vi "Json_Data_Path.vi"(2 "Json File Path":path, 7 "ERD Data Out":cluster{"ERD Number":u16, "Data":string}[](array[cluster]) {"ERD Number" format="%.0x"}, 11 "error in":errorcluster) -> (6 "Array":T1(array[cluster]) {"ERD Number" format="%x"}, 15 "error out":errorcluster)   [LabVIEW 2021]
uses:
  <vilib>/JDP Science/JSONtext/String Subset.vi
  <vilib>/JDP Science/JSONtext/support/Strip Quotes and Unescape.vi
  <vilib>/JDP Science/JSONtext/support/Unescape JSON string.vi
  <vilib>/JDP Science/JSONtext/Parsing/Parse Full Path or Item Name.vi
  <vilib>/JDP Science/JSONtext/Offset/Find Item Locations by Path.vi
  <vilib>/JDP Science/JSONtext/JSONtext.lvlib
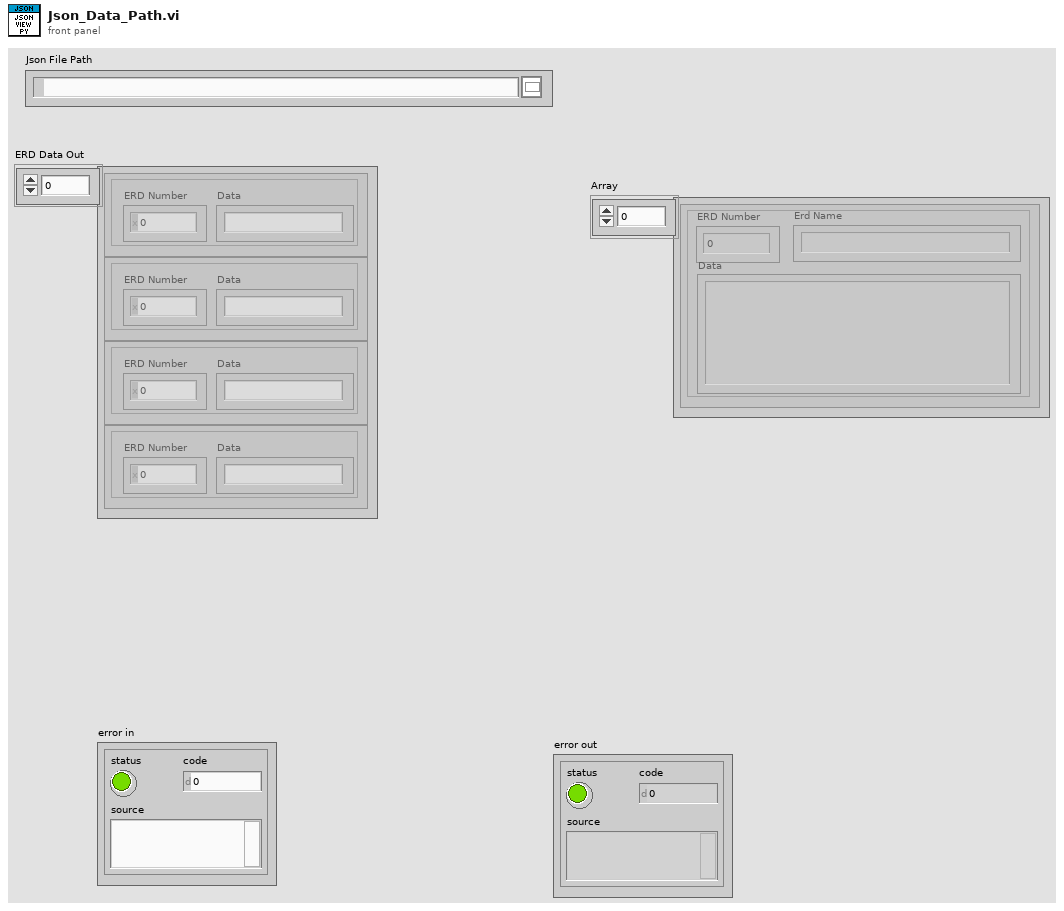
[diagram p1: front panel]
types:
  T1 = cluster{"ERD Number":u16, "Data":string, "Erd Name":string}[]
  T2 = cluster{"ERD Number":u16, "Data":string, "Erd Name":string}
  T3 = enum16{"open", "replace", "create", "open or create", "replace or create", "replace or create with confirmation"}
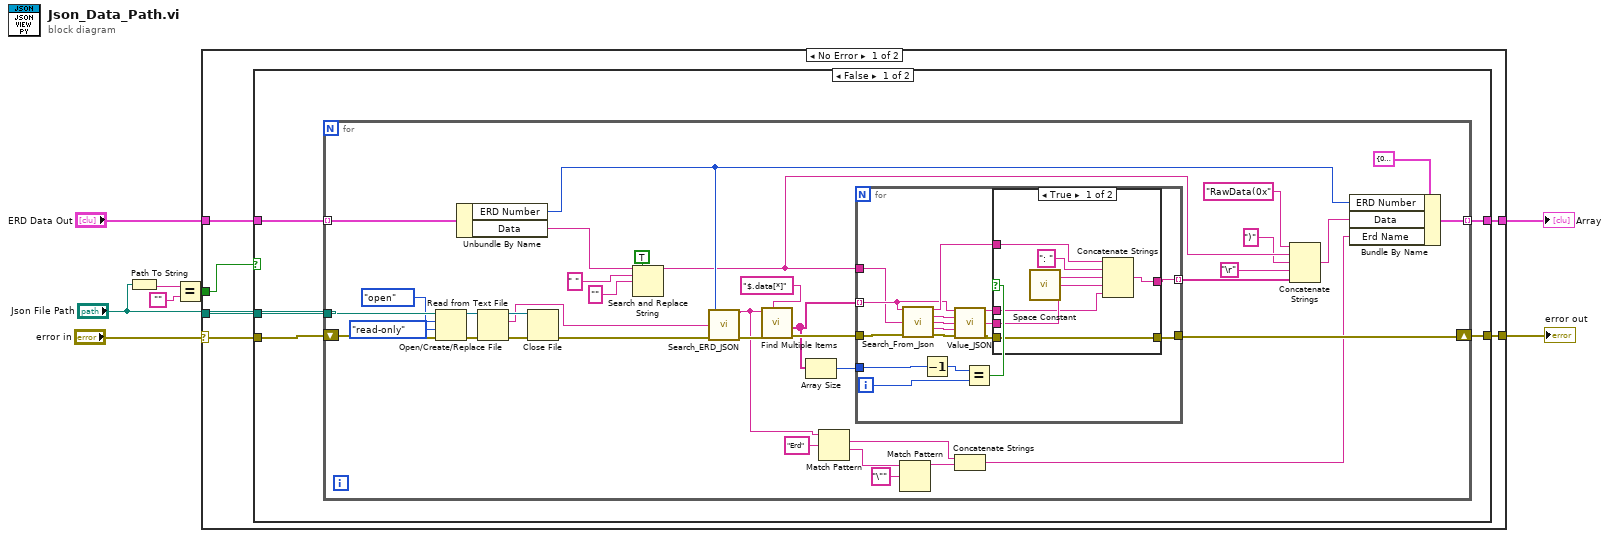
[diagram p0: block diagram]
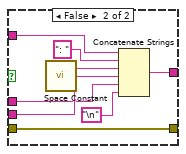
[diagram p2: hidden frame]
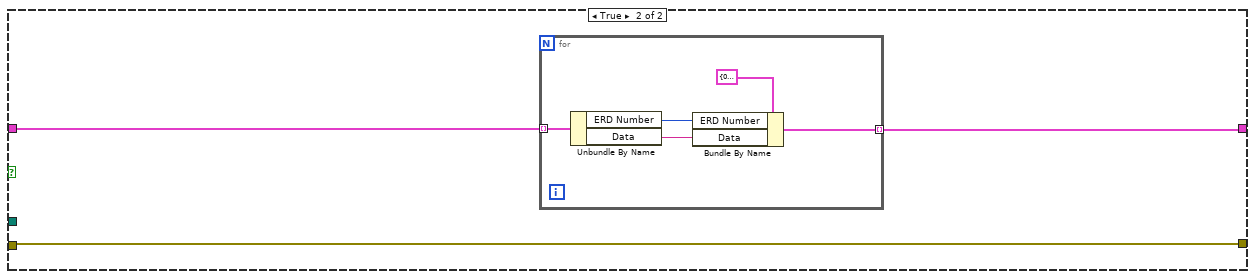
[diagram p3: hidden frame]
diagram:
  n1 = Path To String(path="Json File Path") -> (string=w4:string)
  n2 = Equal?(x=w4, y="") -> (x = y?=w2:bool)
  n3 = case shown="No Error" "error in" {
    selector: "error in" -> [w11 w97]
    tunnel: [w10 w97] -> w7
    tunnel: "Json File Path" -> [w14 _]
    tunnel: "ERD Data Out" -> [w13 _]
    tunnel: [w12 _] -> w1
    tunnel: w2 -> [w9 _]
    frame No Error {
      n4 = case shown="False" w9 {
        tunnel: w14 -> [w19 _]
        tunnel: w13 -> [w16 w90]
        tunnel: [w15 w89] -> w12
        tunnel: w11 -> [w18 w91]
        tunnel: [w17 w91] -> w10
        frame False {
          n5 = for {
            tunnel: w19 -> [w52]
            shift-right: [w41] -> w17
            shift-left: w18 -> [w47]
            tunnel: w16 -> [w36] mode=indexing
            tunnel: [w35] -> w15 mode=indexing
            n6 = Open/Create/Replace File(file path (use dialog)=w52, error in=w47, operation (0:open)=T3."open", access (0:read/write)=enum16{"read/write", "read-only", "write-only"}."read-only") -> (refnum out=w54:refnum<file>, error out=w56:errorcluster)  [unwired: 2 in, 1 out]
            n7 = Unbundle By Name(w36) -> ("ERD Number"=w45:u16, "Data"=w37:string)
            n8 = Read from Text File(file (use dialog)=w54, error in=w56) -> (refnum out=w53:refnum<file>, text=w42:string, error out=w55:errorcluster)  [unwired: 2 in, 1 out]
            n9 = Close File(refnum=w53, error in=w55) -> (error out=w43:errorcluster)  [unwired: 1 out]
            n10 = Search and Replace String(replace all?=TRUE ("replace all? (F)"), input string=w37, search string=" ", replace string="" ("replace string (\"\")")) -> (result string=w31:string)  [unwired: 4 in, 3 out]
            n11 = call "Search_ERD_JSON.vi"("ERD Number"=w45, "JSON Text"=w42, "error in"=w43) -> ("ERD"=w22:string, "error out"=w46:errorcluster)  [unwired: 11 in]
            n12 = call <vilib>:"Find Multiple Items.vi"("$Path or Item Name"="$.data[*]", "error in (no error)"=w46, "JSON"=w22) -> ("error out"=w44:errorcluster, "<JSON>"=w34:string[])  [unwired: 5 in, 2 out]
            n13 = Array Size(array=w34) -> (size(s)=w33:i32)
            n14 = Match Pattern(string=w22, regular expression="Erd") -> (match substring=w23:string, after substring=w26:string)  [unwired: 1 in, 2 out]
            n15 = for {
              tunnel: w34 -> [w71] mode=indexing
              tunnel: w31 -> [w57]
              tunnel: [w73] -> w29 mode=indexing
              tunnel: [w63] -> w41
              tunnel: w44 -> [w66]
              tunnel: w33 -> [w60]
              i -> [w64]
              n16 = call "Search_From_Json.vi"("Data JSON"=w71, "ERD"=w57, "error in"=w66) -> ("Name"=w72:string, "Type"=w70:string, "Size data"=w69:string, "Hexa"=w68:string, "error IO"=w67:errorcluster)  [unwired: 8 in]
              n17 = Decrement(x=w60) -> (x-1=w59:i32)
              n18 = call "Value_JSON.vi"("Data JSON"=w71, "Type"=w70, "Size data"=w69, "Hexa"=w68, "error in"=w67) -> ("Value_string"=w58:string, "Hexa value"=w65:string, "error IO"=w62:errorcluster)  [unwired: 8 in]
              n19 = Equal?(x=w59, y=w64) -> (x = y?=w61:bool)
              n20 = case shown="True" w61 {
                tunnel: [w78 w86] -> w73
                tunnel: w72 -> [w77 w85]
                tunnel: w65 -> [w76 w84]
                tunnel: [w75 w83] -> w63
                tunnel: w62 -> [w75 w83]
                tunnel: w58 -> [w74 w81]
                frame True {
                  n21 = call <vilib>:"Space Constant.vi"() -> ("String"=w79:string)
                  n22 = Concatenate Strings(w77, ": " ("string"), w76, w79, w74) -> (w78:string)
                }
                frame False {
                  n23 = call <vilib>:"Space Constant.vi"() -> ("String"=w87:string)
                  n24 = Concatenate Strings(w85, ": " ("string"), w84, w87, w81, "\n") -> (w86:string)
                }
              }
            }
            n25 = Match Pattern(string=w26, regular expression="\"") -> (before substring=w24:string)  [unwired: 1 in, 3 out]
            n26 = Concatenate Strings(w23, w24) -> (w20:string)
            n27 = Concatenate Strings("RawData(0x" ("string"), w31, ")" ("string"), "\r", w29) -> (w38:string)
            n28 = Bundle By Name(cluster=T2 {"ERD Number"=0, "Data"="", "Erd Name"=""} ("ERD Output"), "ERD Number"=w45, "Data"=w38, "Erd Name"=w20) -> (w35:T2)
          }
        }
        frame True {
          n29 = for {
            tunnel: w90 -> [w96] mode=indexing
            tunnel: [w92] -> w89 mode=indexing
            n30 = Unbundle By Name(w96) -> ("ERD Number"=w94:u16, "Data"=w93:string)
            n31 = Bundle By Name(cluster=T2 {"ERD Number"=0, "Data"="", "Erd Name"=""} ("ERD Output"), "ERD Number"=w94, "Data"=w93) -> (w92:T2)
          }
        }
      }
    }
    frame Error {
    }
  }
  "error out" <- w7
  "Array" <- w1
